vi "iHR550 Correct Center v10.5.0.vi"(1 "Set?":bool=TRUE, 2 "Description":string="1", 3 "Position In (nm)":dbl=897.9988) -> (0 "Position Out (nm)":dbl=897.9988)   [LabVIEW 2010]
uses:
  <vilib>/Utility/config.llb/Read Key (Double).vi
  <vilib>/Utility/config.llb/NI_LVConfig.lvlib
panel:
  in  "Config Name":string="iHR550 Coefficients 210915"
  out "Error Out":errorcluster
  in  "Error In":errorcluster
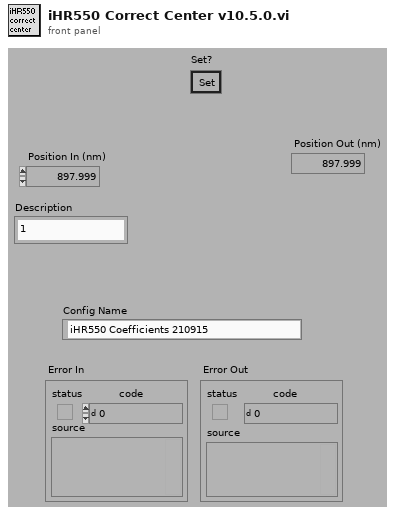
[diagram p1: front panel]
types:
  T1 = typedef "NI_LVConfig.lvlib/Config Data RefNum.ctl" = refnum<k1>
  T2 = cluster{"[0]":dbl, "[1]":dbl, "[2]":dbl, "[3]":dbl}
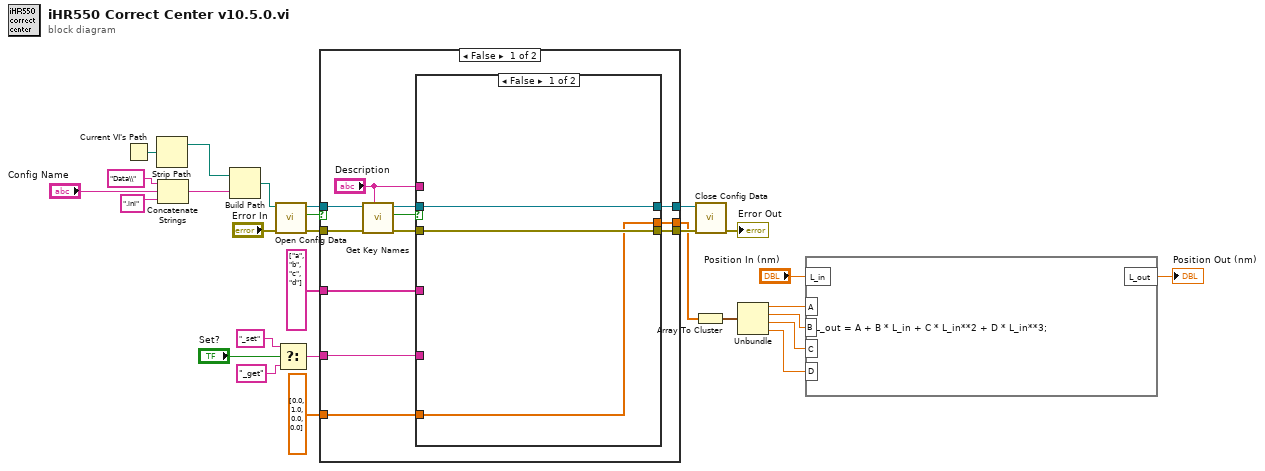
[diagram p0: block diagram]
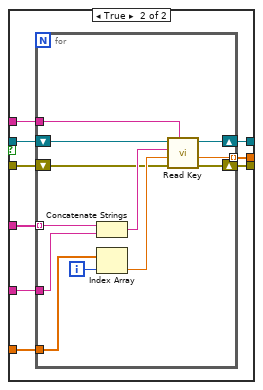
[diagram p2: hidden frame]
diagram:
  n1 = Current VI's Path() -> (path=w2:path)
  n2 = Strip Path(path=w2) -> (stripped path=w1:path)  [unwired: 1 out]
  n3 = Concatenate Strings("Data\\" ("name or relative path"), "Config Name", ".ini" ("name or relative path")) -> (w4:string)
  n4 = Build Path(base path=w1, name or relative path=w4) -> (appended path=w3:path)
  n5 = call <vilib>:"Open Config Data.vi"("error in (no error)"="Error In", "configuration file path"=w3) -> ("error out"=w23:errorcluster, "file created?"=w25:bool, "refnum"=w24:T1)  [unwired: 7 in]
  n6 = Select(t="_set", s="Set?", f="_get") -> (s? t:f=w8:string)
  n7 = case shown="False" w25 {
    tunnel: w24 -> [w40 w66]
    tunnel: w23 -> [w39 w67]
    tunnel: [w34 w67] -> w22
    tunnel: [w33 w66] -> w20
    tunnel: [w32 w65] -> w17
    tunnel: dbl[] [0.0, 1.0, 0.0, 0.0] -> [w31 w65]
    tunnel: string[] ["a", "b", "c", "d"] -> [w30 _]
    tunnel: w8 -> [w29 _]
    frame False {
      n8 = call <vilib>:"Get Key Names.vi"("section"="Description", "error in (no error)"=w39, "refnum"=w40) -> ("error out"=w35:errorcluster, "section exists?"=w38:bool, "refnum out"=w37:T1)  [unwired: 5 in, 1 out]
      n9 = case shown="False" w38 {
        tunnel: w37 -> [w43 w46]
        tunnel: "Description" -> [_ w52]
        tunnel: w35 -> [w42 w45]
        tunnel: [w42 w51] -> w34
        tunnel: [w43 w50] -> w33
        tunnel: [w41 w49] -> w32
        tunnel: w31 -> [w41 w48]
        tunnel: w30 -> [_ w47]
        tunnel: w29 -> [_ w44]
        frame False {
        }
        frame True {
          n10 = for {
            tunnel: w52 -> [w64]
            tunnel: w47 -> [w62] mode=indexing
            tunnel: w44 -> [w63]
            tunnel: w48 -> [w57]
            shift-right: [w60] -> w51
            shift-left: w45 -> [w53]
            shift-right: [w59] -> w50
            shift-left: w46 -> [w54]
            tunnel: [w58] -> w49 mode=indexing
            i -> [w55]
            n11 = Concatenate Strings(w62, w63) -> (w61:string)
            n12 = Index Array(array=w57, index=w55) -> (element=w56:dbl)
            n13 = call-poly <vilib>:"Read Key.vi"("section"=w64, "error in (no error)"=w53, "default value"=w56, "key"=w61, "refnum"=w54) -> ("error out"=w60:errorcluster, "value"=w58:dbl, "refnum out"=w59:T1)  [unwired: 3 in, 1 out]
          }
        }
      }
    }
    frame True {
    }
  }
  n14 = Array To Cluster(array=w17) -> (cluster=w16:T2)
  n15 = call <vilib>:"Close Config Data.vi"("error in (no error)"=w22, "refnum"=w20) -> ("error out"=→"Error Out":errorcluster)  [unwired: 8 in, 1 out]
  n16 = Unbundle(w16) -> ("[0]"=w15:dbl, "[1]"=w14:dbl, "[2]"=w13:dbl, "[3]"=w12:dbl)
  n17 = formula code="L_out = A + B * L_in + C * L_in**2 + D * L_in**3;"("L_in"="Position In (nm)", "A"=w15, "B"=w14, "C"=w13, "D"=w12) -> ("L_out"=→"Position Out (nm)":dbl)
